vi "Server.vi"(8 "error in":errorcluster, 10 "port (54444)":u16=54444, 11 "stop notifier":refnum<notifier>) -> (0 "error  out":errorcluster)   [LabVIEW 2016, in "NI_CCC.lvlib"]
uses:
  NI_CCC.lvlib
  FG Server Instances Action.ctl
  Server State.ctl
  <vilib>/NI/STM/TCP/TCP Read Options.ctl
  <vilib>/NI/STM/SubVIs/MetaDataElement.ctl
  <vilib>/NI/Current Value Table/Delete Group.vi
  <vilib>/Utility/error.llb/Clear Errors.vi
  Write Error.vi
  <vilib>/NI/Current Value Table/Write Grouped Tags.vi
  <vilib>/NI/Current Value Table/Read Grouped Tags.vi
  <vilib>/NI/Current Value Table/Write grouped data to tags.vi
  <vilib>/NI/Current Value Table/Read tags into grouped data.vi
  <vilib>/NI/Current Value Table/Write Index Set.vi
  <vilib>/NI/Current Value Table/DataTypes/Double_Write Index Set.vi
  <vilib>/NI/Current Value Table/DataTypes/Array of String_Write Index Set.vi
  <vilib>/NI/Current Value Table/DataTypes/Array of Boolean_Write Index Set.vi
  <vilib>/NI/Current Value Table/DataTypes/Array of Single_Write Index Set.vi
  <vilib>/NI/Current Value Table/DataTypes/Array of Double_Write Index Set.vi
  <vilib>/NI/Current Value Table/DataTypes/Array of I8_Write Index Set.vi
  <vilib>/NI/Current Value Table/DataTypes/Array of I16_Write Index Set.vi
  <vilib>/NI/Current Value Table/DataTypes/Array of I32_Write Index Set.vi
  <vilib>/NI/Current Value Table/DataTypes/Array of I64_Write Index Set.vi
  <vilib>/NI/Current Value Table/DataTypes/Array of U64_Write Index Set.vi
  <vilib>/NI/Current Value Table/DataTypes/Array of U32_Write Index Set.vi
  <vilib>/NI/Current Value Table/DataTypes/Array of U16_Write Index Set.vi
  <vilib>/NI/Current Value Table/DataTypes/Array of U8_Write Index Set.vi
  <vilib>/NI/Current Value Table/DataTypes/Boolean_Write Index Set.vi
  <vilib>/NI/Current Value Table/DataTypes/String_Write Index Set.vi
  <vilib>/NI/Current Value Table/DataTypes/U8_Write Index Set.vi
  <vilib>/NI/Current Value Table/DataTypes/U16_Write Index Set.vi
  <vilib>/NI/Current Value Table/DataTypes/U32_Write Index Set.vi
  <vilib>/NI/Current Value Table/DataTypes/U64_Write Index Set.vi
  <vilib>/NI/Current Value Table/DataTypes/I8_Write Index Set.vi
  <vilib>/NI/Current Value Table/DataTypes/I16_Write Index Set.vi
  <vilib>/NI/Current Value Table/DataTypes/I32_Write Index Set.vi
  <vilib>/NI/Current Value Table/DataTypes/I64_Write Index Set.vi
  <vilib>/NI/Current Value Table/DataTypes/Single_Write Index Set.vi
  <vilib>/NI/Current Value Table/Read Index Set.vi
  <vilib>/NI/Current Value Table/DataTypes/Double_Read Index Set.vi
  <vilib>/NI/Current Value Table/DataTypes/Array of String_Read Index Set.vi
  <vilib>/NI/Current Value Table/DataTypes/Array of Boolean_Read Index Set.vi
  <vilib>/NI/Current Value Table/DataTypes/Array of Single_Read Index Set.vi
  <vilib>/NI/Current Value Table/DataTypes/Array of Double_Read Index Set.vi
  <vilib>/NI/Current Value Table/DataTypes/Array of I8_Read Index Set.vi
  <vilib>/NI/Current Value Table/DataTypes/Array of I16_Read Index Set.vi
  <vilib>/NI/Current Value Table/DataTypes/Array of I32_Read Index Set.vi
  <vilib>/NI/Current Value Table/DataTypes/Array of I64_Read Index Set.vi
  <vilib>/NI/Current Value Table/DataTypes/Array of U64_Read Index Set.vi
  <vilib>/NI/Current Value Table/DataTypes/Array of U32_Read Index Set.vi
  <vilib>/NI/Current Value Table/DataTypes/Array of U16_Read Index Set.vi
  <vilib>/NI/Current Value Table/DataTypes/Array of U8_Read Index Set.vi
  <vilib>/NI/Current Value Table/DataTypes/Boolean_Read Index Set.vi
  <vilib>/NI/Current Value Table/DataTypes/String_Read Index Set.vi
  <vilib>/NI/Current Value Table/DataTypes/U8_Read Index Set.vi
  <vilib>/NI/Current Value Table/DataTypes/U16_Read Index Set.vi
  <vilib>/NI/Current Value Table/DataTypes/U32_Read Index Set.vi
  <vilib>/NI/Current Value Table/DataTypes/U64_Read Index Set.vi
  <vilib>/NI/Current Value Table/DataTypes/I8_Read Index Set.vi
  <vilib>/NI/Current Value Table/DataTypes/I16_Read Index Set.vi
  <vilib>/NI/Current Value Table/DataTypes/I32_Read Index Set.vi
  <vilib>/NI/Current Value Table/DataTypes/I64_Read Index Set.vi
  <vilib>/NI/Current Value Table/DataTypes/Single_Read Index Set.vi
  <vilib>/NI/STM/TCP/Write Message (TCP).vi
  <vilib>/NI/Current Value Table/Memory Block.vi
  <vilib>/NI/Current Value Table/DataTypes/Single_Memory Block.vi
  <vilib>/NI/Current Value Table/DataTypes/I64_Memory Block.vi
  <vilib>/NI/Current Value Table/DataTypes/I32_Memory Block.vi
  <vilib>/NI/Current Value Table/DataTypes/I16_Memory Block.vi
  <vilib>/NI/Current Value Table/DataTypes/I8_Memory Block.vi
  <vilib>/NI/Current Value Table/DataTypes/U64_Memory Block.vi
  <vilib>/NI/Current Value Table/DataTypes/U32_Memory Block.vi
  <vilib>/NI/Current Value Table/DataTypes/U16_Memory Block.vi
  <vilib>/NI/Current Value Table/DataTypes/U8_Memory Block.vi
  <vilib>/NI/Current Value Table/DataTypes/String_Memory Block.vi
  <vilib>/NI/Current Value Table/DataTypes/Boolean_Memory Block.vi
  <vilib>/NI/Current Value Table/DataTypes/Array of U8_Memory Block.vi
  <vilib>/NI/Current Value Table/DataTypes/Array of U16_Memory Block.vi
  <vilib>/NI/Current Value Table/DataTypes/Array of U32_Memory Block.vi
  <vilib>/NI/Current Value Table/DataTypes/Array of U64_Memory Block.vi
  <vilib>/NI/Current Value Table/DataTypes/Array of I64_Memory Block.vi
  <vilib>/NI/Current Value Table/DataTypes/Array of I32_Memory Block.vi
  <vilib>/NI/Current Value Table/DataTypes/Array of I16_Memory Block.vi
  <vilib>/NI/Current Value Table/DataTypes/Array of I8_Memory Block.vi
  <vilib>/NI/Current Value Table/DataTypes/Array of Double_Memory Block.vi
  <vilib>/NI/Current Value Table/DataTypes/Array of Single_Memory Block.vi
  <vilib>/NI/Current Value Table/DataTypes/Array of Boolean_Memory Block.vi
  <vilib>/NI/Current Value Table/DataTypes/Array of String_Memory Block.vi
  <vilib>/NI/Current Value Table/DataTypes/Double_Memory Block.vi
  <vilib>/NI/Current Value Table/FGVs/Group Memory.vi
  Configure Server Group.vi
  <vilib>/NI/STM/TCP/Write Meta Data (TCP Clst).vi
  <vilib>/NI/STM/NI STM.lvlib
panel:
  in  "stop":bool
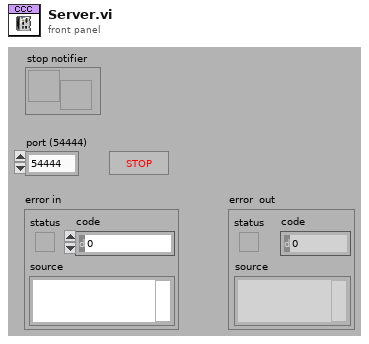
[diagram p1: front panel]
types:
  T1 = typedef "NI_CCC.lvlib/FG Server Instances Action.ctl" = enum16{"Find Instance", "Find All", "Register Instance", "Unregister Instance", "Unregister All"}
  T2 = typedef "NI_CCC.lvlib/Server State.ctl" = cluster{"write group name":string, "read group name":string, "write tags exist":bool, "read tags exist":bool}
  T3 = typedef "NI STM.lvlib/MetaDataElement.ctl" = string
  T4 = typedef "NI STM.lvlib/TCP Read Options.ctl" = cluster{"ignore timeout error":bool, "timeout ms (1000)":i32}
  T5 = typedef "NI_CCC.lvlib/Server Instance Data.ctl" = cluster{"server ref":refnum<vi>, "stop notifier":refnum<notifier>}
  T6 = typedef "NI STM.lvlib/TCP Connection Info.ctl" = cluster{"connection ID":refnum<k5>, "meta data":T3[]}
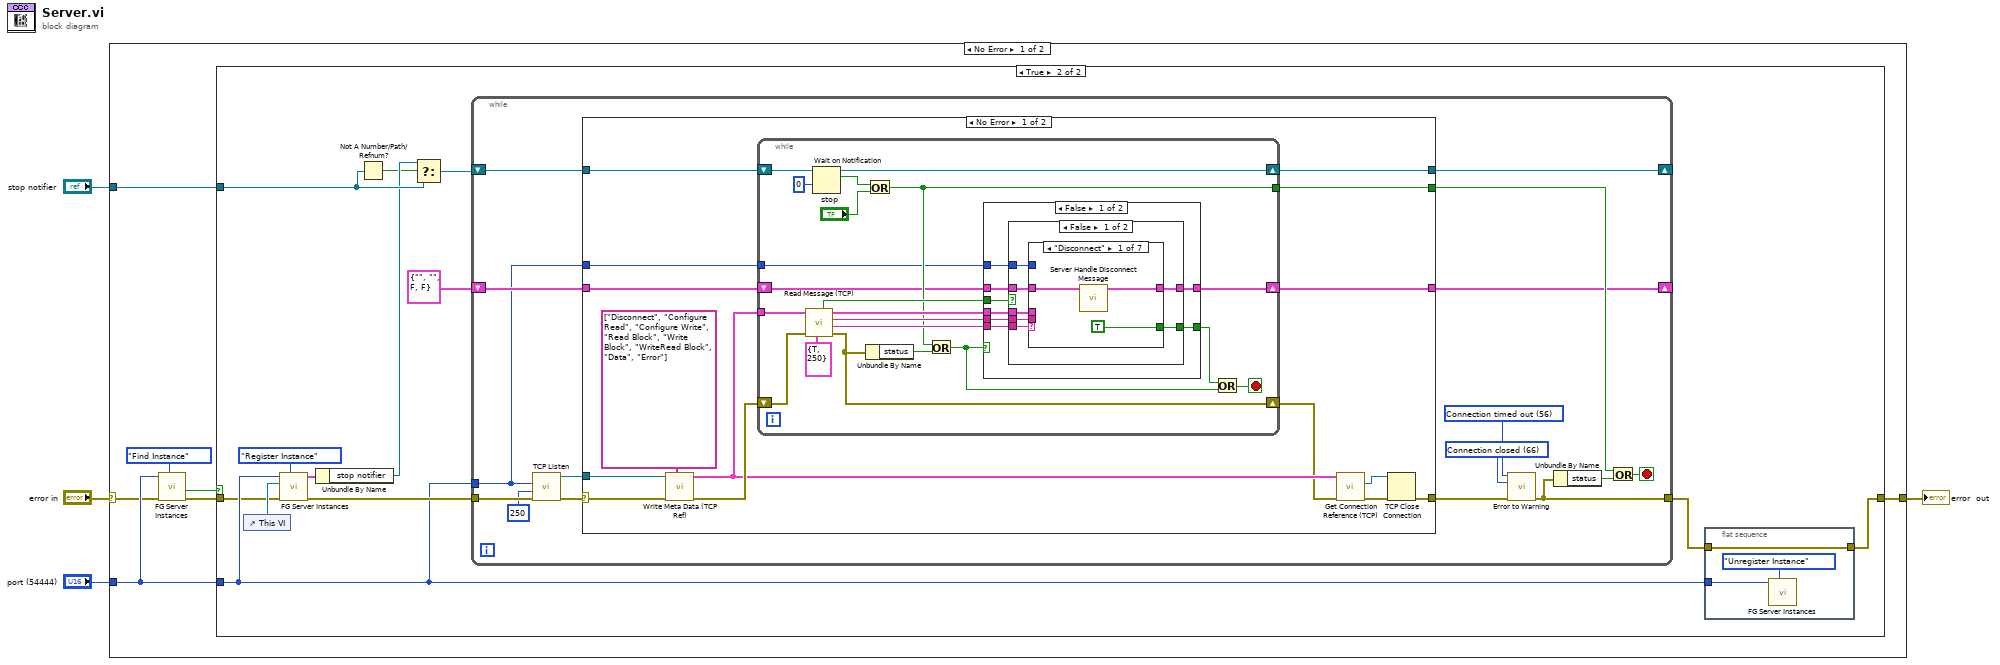
[diagram p0: block diagram]
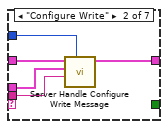
[diagram p3: hidden frame]
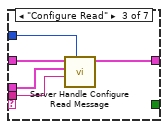
[diagram p4: hidden frame]
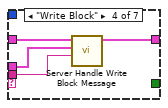
[diagram p5: hidden frame]
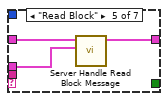
[diagram p6: hidden frame]
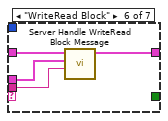
[diagram p7: hidden frame]
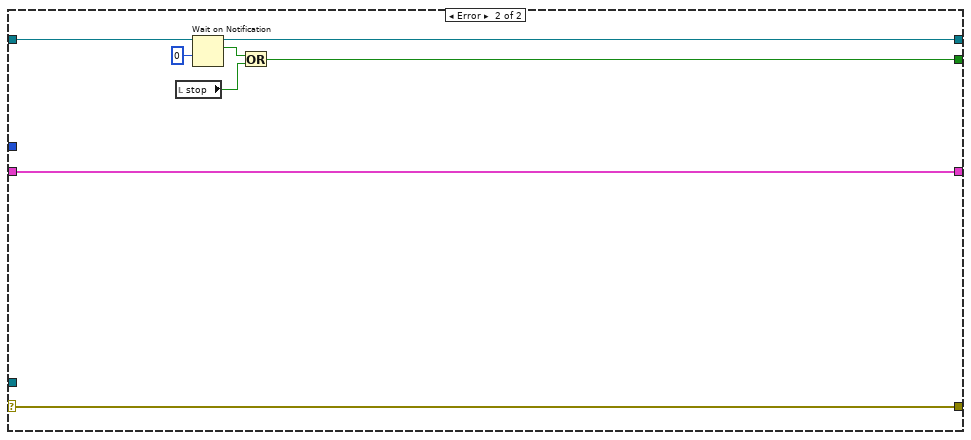
[diagram p11: hidden frame]
diagram:
  n1 = case shown="No Error" "error in" {
    selector: "error in" -> [w5 w131]
    tunnel: "stop notifier" -> [w11 _]
    tunnel: [w10 w131] -> w3
    tunnel: "port (54444)" -> [w8 _]
    frame No Error {
      n2 = call "FG Server Instances.vi"("action"=FG_Server_Instances_Action."Find Instance", "error in"=w5, "port"=w8) -> ("error out"=w7:errorcluster, "failed?"=w6:bool)  [unwired: 5 in, 2 out]
      n3 = case shown="True" w6 {
        tunnel: w11 -> [_ w18]
        tunnel: [w12 w21] -> w10
        tunnel: w8 -> [_ w20]
        tunnel: w7 -> [w12 w19]
        frame False {
          # "There is already another instance of Server.vi using this port."
        }
        frame True {
          n4 = control-ref of="This VI"() -> (w24:refnum<vi>)
          n5 = call "FG Server Instances.vi"("action"=FG_Server_Instances_Action."Register Instance", "error in"=w19, "server refnum in"=w24, "port"=w20) -> ("error out"=w23:errorcluster, "server instance"=w16:T5)  [unwired: 4 in, 2 out]
          n6 = Unbundle By Name(w16) -> ("stop notifier"=w15:refnum<notifier>)
          n7 = Not A Number/Path/Refnum?(number/path/refnum=w18) -> (NaN/Path/Refnum?=w14:bool)
          n8 = Select(t=w15, s=w14, f=w18) -> (s? t:f=w17:refnum<notifier>)
          n9 = while {
            tunnel: [w34] -> w22
            tunnel: w23 -> [w43]
            shift-right: [w32] -> _
            shift-left: w17 -> [w33]
            shift-right: [w30] -> _
            shift-left: T2 {"write group name"="", "read group name"="", "write tags exist"=FALSE, "read tags exist"=FALSE} ("state") -> [w31]
            tunnel: w20 -> [w29]
            stop <- w40 stop-if-true
            w37 = 56 items=["No Error", "Argument Error", "Memory Full", "Out of Zone", "End of File", "File Already Open", "Generic File IO Error", "File Not Found", "File Permission Error", "Disk Full", "Duplicate Path", "Too Many Files Open", "Not Enabled", "Resource File Not Found", "Cannot Add Resource", "Resource Not Found", "Image Not Found", "Image Memory Error", "Pen Does Not Exist", "Config Bad Type", "Config Token Not Found", "Config Parse Error", "Config Memory Error", "Bad External Code Format", "Bad External Code Offset", "External Code Not Present", "Null Window", "Destroy Window Mixup", "Null Menu", "Print Aborted", "Bad Print Record", "Print Driver Error", "Windows Error During Print", "Memory Error During Print", "Print Dialog Error", "Generic Print Error", "Invalid Device Refnum", "Device Not Found", "Device Parameter Error", "Device Unit Error", "Can't Open Device", "Device Call Aborted", "Generic Error", "Cancelled By User", "Object ID Too Low", "Object ID Too High", "Object Not In Heap", "Unknown Heap", "Bad DefProc ID", "DefProc Not In Table", "Message Out Of Range", "Null Method", "Unknown Message", "Manager Call Not Supported", "Bad address", "Connection In progress", "Connection timed out", "Connection is already in progress", "Network attribute not supported", "Network error", "Address in use", "System out of memory", "Connection aborted", "Connection refused", "Connection is not connected", "Connection is already connected", "Connection closed", "Initialize error (interapplication manager)", "Bad occurrence", "Wait on unbound occurrence handler", "Occurrence queue overflow", "Bad path", "Semaphore not signaled", "Unrecognized type (interapplication manager)"] ("2nd Error to Convert")
            w36 = 66 items=["No Error", "Argument Error", "Memory Full", "Out of Zone", "End of File", "File Already Open", "Generic File IO Error", "File Not Found", "File Permission Error", "Disk Full", "Duplicate Path", "Too Many Files Open", "Not Enabled", "Resource File Not Found", "Cannot Add Resource", "Resource Not Found", "Image Not Found", "Image Memory Error", "Pen Does Not Exist", "Config Bad Type", "Config Token Not Found", "Config Parse Error", "Config Memory Error", "Bad External Code Format", "Bad External Code Offset", "External Code Not Present", "Null Window", "Destroy Window Mixup", "Null Menu", "Print Aborted", "Bad Print Record", "Print Driver Error", "Windows Error During Print", "Memory Error During Print", "Print Dialog Error", "Generic Print Error", "Invalid Device Refnum", "Device Not Found", "Device Parameter Error", "Device Unit Error", "Can't Open Device", "Device Call Aborted", "Generic Error", "Cancelled By User", "Object ID Too Low", "Object ID Too High", "Object Not In Heap", "Unknown Heap", "Bad DefProc ID", "DefProc Not In Table", "Message Out Of Range", "Null Method", "Unknown Message", "Manager Call Not Supported", "Bad address", "Connection In progress", "Connection timed out", "Connection is already in progress", "Network attribute not supported", "Network error", "Address in use", "System out of memory", "Connection aborted", "Connection refused", "Connection is not connected", "Connection is already connected", "Connection closed", "Initialize error (interapplication manager)", "Bad occurrence", "Wait on unbound occurrence handler", "Occurrence queue overflow", "Bad path", "Semaphore not signaled", "Unrecognized type (interapplication manager)"] ("1st Error to Convert")
            n10 = call <vilib>:"TCP Listen.vi"("error in (no error)"=w43, "timeout ms (wait forever: -1)"=250, "port"=w29) -> ("error out"=w38:errorcluster, "connection ID"=w44:refnum<k5>)  [unwired: 1 in, 6 out]
            n11 = case shown="No Error" w38 {
              selector: w38 -> [w56 w130]
              tunnel: w44 -> [w59 _]
              tunnel: [w49 w130] -> w35
              tunnel: [w57 w124] -> w39
              tunnel: w33 -> [w51 w128]
              tunnel: [w50 w127] -> w32
              tunnel: w31 -> [w48 w123]
              tunnel: [w47 w123] -> w30
              tunnel: w29 -> [w45 _]
              frame No Error {
                n12 = call <vilib>:"Write Meta Data (TCP Ref).vi"("meta data"=T3[] ["Disconnect", "Configure Read", "Configure Write", "Read Block", "Write Block", "WriteRead Block", "Data", "Error"] ("Meta data"), "error in"=w56, "connection ID"=w59) -> ("error out"=w55:errorcluster, "connection info out"=w53:T6)  [unwired: 7 in]
                n13 = while {
                  tunnel: w53 -> [w72]
                  tunnel: [w67] -> w57
                  shift-right: [w66] -> w50
                  shift-left: w51 -> [w71]
                  shift-right: [w64] -> w47
                  shift-left: w48 -> [w65]
                  shift-right: [w74] -> w46
                  shift-left: w55 -> [w80]
                  tunnel: w45 -> [w60]
                  stop <- w62 stop-if-true
                  n14 = call <vilib>:"Read Message (TCP).vi"("options"=T4 {"ignore timeout error"=TRUE, "timeout ms (1000)"=250} ("Options"), "error in"=w80, "connection info in"=w72) -> ("error out"=w74:errorcluster, "name"=w79:T3, "data string"=w78:string, "connection info out"=w75:T6, "timed out?"=w76:bool)  [unwired: 3 in, 1 out]
                  n15 = Wait on Notification(notifier=w71, timeout in ms (-1)=0) -> (notifier out=w66:refnum<notifier>, notification=w69:bool)  [unwired: 2 in, 2 out]
                  n16 = Unbundle By Name(w74) -> ("status"=w77:bool)
                  n17 = Or(x=w69, y="stop") -> (x .or. y?=w67:bool)
                  n18 = Or(x=w67, y=w77) -> (x .or. y?=w61:bool)
                  n19 = case shown="False" w61 {
                    tunnel: w79 -> [w88 _]
                    tunnel: w78 -> [w87 _]
                    tunnel: w76 -> [w86 _]
                    tunnel: w75 -> [w85 _]
                    tunnel: w65 -> [w84 w122]
                    tunnel: [w83 w122] -> w64
                    tunnel: [w82 _] -> w63
                    tunnel: w60 -> [w81 _]
                    frame False {
                      n20 = case shown="False" w86 {
                        tunnel: w88 -> [w93 _]
                        tunnel: w87 -> [w95 _]
                        tunnel: w85 -> [w94 _]
                        tunnel: w84 -> [w92 w121]
                        tunnel: [w91 w121] -> w83
                        tunnel: [w90 _] -> w82
                        tunnel: w81 -> [w89 _]
                        frame False {
                          n21 = case shown="\"Disconnect\"" w93 {
                            tunnel: w95 -> [_ w100 w105 w110 _ w116 _]
                            tunnel: w94 -> [_ w101 w106 w111 w113 w117 _]
                            tunnel: w92 -> [w97 w103 w108 w112 w115 w119 w120]
                            tunnel: [w96 w102 w107 w109 w114 w118 w120] -> w91
                            tunnel: [TRUE _ _ _ _ _ _] -> w90
                            tunnel: w89 -> [_ w99 w104 _ _ _ _]
                            frame "Disconnect" {
                              n22 = call "Server Handle Disconnect Message.vi"("state in"=w97) -> ("state out"=w96:T2)  [unwired: 9 in, 1 out]
                            }
                            frame "Configure Write" {
                              n23 = call "Server Handle Configure Write Message.vi"("port"=w99, "data string"=w100, "connection info in"=w101, "state in"=w103) -> ("state out"=w102:T2)  [unwired: 6 in, 1 out]
                            }
                            frame "Configure Read" {
                              n24 = call "Server Handle Configure Read Message.vi"("port"=w104, "data string"=w105, "connection info in"=w106, "state in"=w108) -> ("state out"=w107:T2)  [unwired: 6 in, 1 out]
                            }
                            frame "Write Block" {
                              n25 = call "Server Handle Write Block Message.vi"("data string"=w110, "connection info in"=w111, "state in"=w112) -> ("state out"=w109:T2)  [unwired: 7 in, 1 out]
                            }
                            frame "Read Block" {
                              n26 = call "Server Handle Read Block Message.vi"("connection info in"=w113, "state in"=w115) -> ("state out"=w114:T2)  [unwired: 8 in, 1 out]
                            }
                            frame "WriteRead Block" {
                              n27 = call "Server Handle WriteRead Block Message.vi"("data string"=w116, "connection info in"=w117, "state in"=w119) -> ("state out"=w118:T2)  [unwired: 7 in, 1 out]
                            }
                            frame Default {
                              # "Unhandled Command"
                            }
                          }
                        }
                        frame True {
                        }
                      }
                    }
                    frame True {
                    }
                  }
                  n28 = Or(x=w63, y=w61) -> (x .or. y?=w62:bool)
                }
                n29 = call <vilib>:"Get Connection Reference (TCP).vi"("error in"=w46, "connection info in"=w53) -> ("error out"=w54:errorcluster, "connection ID out"=w52:refnum<k5>)  [unwired: 7 in, 1 out]
                n30 = TCP Close Connection(connection ID=w52, error in (no error)=w54) -> (error out=w49:errorcluster)  [unwired: 2 out]
              }
              frame Error {
                n31 = local read "stop"() -> (w125:bool)
                n32 = Wait on Notification(notifier=w128, timeout in ms (-1)=0) -> (notifier out=w127:refnum<notifier>, notification=w126:bool)  [unwired: 2 in, 2 out]
                n33 = Or(x=w126, y=w125) -> (x .or. y?=w124:bool)
              }
            }
            n34 = call <vilib>:"Error to Warning.vi"("1st Error to Convert"=w37, "2nd Error to Convert"=w36, "error in"=w35) -> ("warning out"=w34:errorcluster)  [unwired: 2 in, 10 out]
            n35 = Unbundle By Name(w34) -> ("status"=w41:bool)
            n36 = Or(x=w39, y=w41) -> (x .or. y?=w40:bool)
          }
          n37 = flat-sequence {
            tunnel: w20 -> [w28]
            tunnel: w22 -> [w26]
            tunnel: [w26] -> w21
            frame #0 {
              n38 = call "FG Server Instances.vi"("action"=FG_Server_Instances_Action."Unregister Instance", "port"=w28) -> ()  [unwired: 6 in, 4 out]
            }
          }
        }
      }
    }
    frame Error {
    }
  }
  "error  out" <- w3
